vi "Ctor.vi"(8 "error in (no error)":errorcluster, 11 "Step in":refnum<class "Step.lvclass">) -> (0 "error out":errorcluster, 3 "Step out":refnum<class "Step.lvclass">)   [LabVIEW 2020, in "TSnax.lvlib" / "Step.lvclass"]
uses:
  Step.lvclass
  Step.lvclass/Step.ctl
  PropertyObject/PropertyObject.lvclass
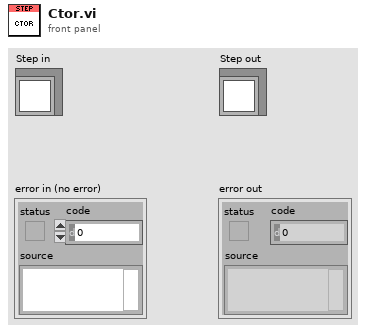
[diagram p1: front panel]
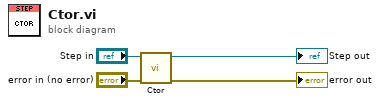
[diagram p0: block diagram]
diagram:
  n1 = call-parent "Ctor.vi"("error in (no error)"="error in (no error)", "PropertyObject in"="Step in") -> ("error out"=→"error out":errorcluster, "PropertyObject out"=→"Step out":refnum<class "Step.lvclass">)  [unwired: 8 in]
